vi "Test Strict Find Items as LV Type1.vi"(11 "Test Case In":refnum<class "Test Strict Find Items as LV Type.lvclass">) -> (0 "error out":errorcluster, 3 "Test Case Out":refnum<class "Test Strict Find Items as LV Type.lvclass">)   [LabVIEW 2023, in "Test Strict Find Items as LV Type.lvclass"]
uses:
  Test Strict Find Items as LV Type.lvclass
  <vilib>/Astemes/LUnit/Test Case.lvclass/Test Case.ctl
  7860c969-8ea9-4e34-a02d-68fc78db45ce.vi
  4993e8ee-a06a-463a-9684-69129f64d5ce.vi
  7860c969-8ea9-4e34-a02d-68fc78db45ce.vi/a4169a97-72fc-4003-a778-603cf20cafa0.vi
  <vilib>/Astemes/LUnit/Append Pass Result.vi
  <vilib>/Astemes/LUnit/Append Fail Result.vi
  <vilib>/Astemes/LUnit/Describe Comparison.vi
  <vilib>/Astemes/LUnit/Compare Variants.vi
  <vilib>/JDP Science/JSONtext/Find Item.vi
  <vilib>/Astemes/LUnit/Run In UI.vi
  <vilib>/JDP Science/JSONtext/Next JSON Value.vi
  <vilib>/JDP Science/JSONtext/String Subset.vi
  <vilib>/Utility/error.llb/Clear Errors.vi
  <vilib>/JDP Science/JSONtext/Parsing/Advance past next JSON Value (inlined COPY).vi
  <vilib>/JDP Science/JSONtext/Parsing/Advance past whitespace.vi
  <vilib>/JDP Science/JSONtext/Parsing/Advance past String.vi
  <vilib>/JDP Science/JSONtext/Parsing/Advance past Number.vi
  <vilib>/JDP Science/JSONtext/Parsing/Advance past Line Ending.vi
  <vilib>/JDP Science/JSONtext/Parsing/Parse Full Path or Item Name.vi
  <vilib>/JDP Science/JSONtext/Parsing/Advance past Array.vi
  <vilib>/JDP Science/JSONtext/Parsing/Advance past Object.vi
  <vilib>/JDP Science/JSONtext/support/Error Cluster From Code.vi
  <vilib>/JDP Science/JSONtext/Offset/Find Item Locations by Path.vi
  <vilib>/JDP Science/JSONtext/JSON text to Variant.vi
  <vilib>/Utility/error.llb/Error Cluster From Error Code.vi
  <vilib>/Astemes/LUnit/Describe Variant.vi
  <vilib>/JDP Science/JSONtext/LVClass Serializer/JSONtext LVClass Serializer.lvclass
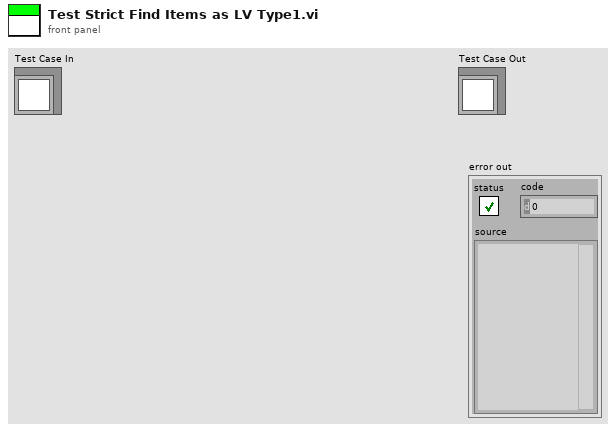
[diagram p1: front panel]
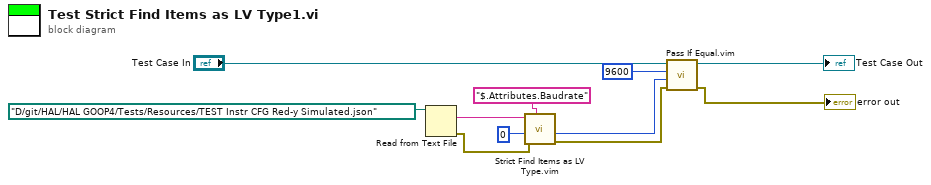
[diagram p0: block diagram]
diagram:
  n1 = Read from Text File(file (use dialog)=path "D:/git/HAL/HAL GOOP4/Tests/Resources/TEST Instr CFG Red-y Simulated.json") -> (text=w7:string, error out=w1:errorcluster)  [unwired: 3 in, 2 out]
  n2 = call "Strict Find Items as LV Type.vim"("$Path or Item Name"="$.Attributes.Baudrate", "error in"=w1, "Data Type and Default Value"=u16 0, "<JSON>"=w7) -> ("error out"=w3:errorcluster, "Data out"=w4:u16)  [unwired: 5 in, 1 out]
  n3 = call "Pass If Equal.vim"("error in (no error)"=w3, "Actual"=w4, "Expected"=u16 9600, "LUnit Test Case In"="Test Case In") -> ("error out"=→"error out":errorcluster, "LUnit Test Case Out"=→"Test Case Out":refnum<class "Test Strict Find Items as LV Type.lvclass">)  [unwired: 6 in]
